vi "Recording Stop Watch.vi"() -> ()   [LabVIEW 2014]
panel:
  out "no message":bool
  in  "Clock Time":u32
  out "Start recording":bool
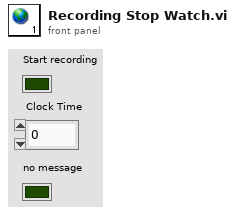
[diagram p1: front panel]
diagram:
